vi "Close shutter.vi"(8 "error in (no error)":errorcluster, 11 "ImageStack in":refnum<class "ImageStack.lvclass">) -> (0 "error out":errorcluster, 3 "ImageStack out":refnum<class "ImageStack.lvclass">)   [LabVIEW 2012, in "ImageStack.lvclass"]
uses:
  ImageStack.lvclass
  <vilib>/Distrio/Murmex/GenericMessage/GenericMessage.lvclass
  <vilib>/Distrio/Murmex/Message/Add or replace parameter.vi
  <vilib>/Distrio/Murmex/Murmex/Murmex.lvclass
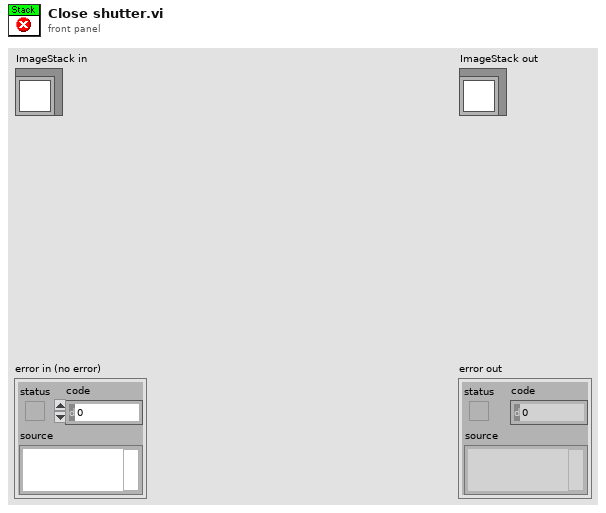
[diagram p1: front panel]
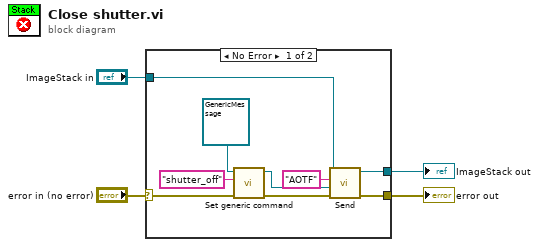
[diagram p0: block diagram]
diagram:
  n1 = case shown="No Error" "error in (no error)" {
    selector: "error in (no error)" -> [w8 w15]
    tunnel: [w7 w15] -> w3
    tunnel: [w5 w14] -> w1
    tunnel: "ImageStack in" -> [w6 w14]
    frame No Error {
      n2 = call <vilib>:"Set generic command.vi"("error in (no error)"=w8, "generic command"="shutter_off", "GenericMessage in"=refnum<class "GenericMessage.lvclass"> refnum ("Distrio Murmex 1.1:GenericMessage")) -> ("error out"=w9:errorcluster, "GenericMessage out"=w11:refnum<class "GenericMessage.lvclass">)  [unwired: 7 in]
      n3 = call <vilib>:"Send.vi"("error in (no error)"=w9, "Message"=w11, "recipient"="AOTF", "Murmex in"=w6) -> ("error out"=w7:errorcluster, "Murmex out"=w5:refnum<class "ImageStack.lvclass">)  [unwired: 6 in]
    }
    frame Error {
    }
  }
  "error out" <- w3
  "ImageStack out" <- w1
